vi "Set Output Voltage.vi"(8 "Error In":errorcluster, 9 "Channel":i32, 10 "Voltage":dbl[unit], 11 "BNT_DAQmx-MCSV in":refnum<class "BNT_DAQmx-MCSV.lvclass">) -> (0 "Error Out":errorcluster, 3 "BNT_DAQmx-MCSV out":refnum<class "BNT_DAQmx-MCSV.lvclass">)   [LabVIEW 2016, in "BNT_DAQmx.lvlib" / "BNT_DAQmx-MCSV.lvclass"]
doc: "Write voltage values to DAQmx device and publish.\n\nTimeout is set to constant 1s."
uses:
  BNT_DAQmx-MCSV.lvclass
  BNT_DAQmx-MCSV.lvclass/BNT_DAQmx-MCSV.ctl
  CSPP_Core/Classes/CS++ProcessVariables/PVConnection/PVConnection.lvclass/PVConnection.ctl
  CSPP_Core/Classes/CS++ProcessVariables/ProcessVariable/PV.lvclass/PV.ctl
  <vilib>/DAQmx/write.llb/DAQmx Write (Analog 1D DBL NChan 1Samp).vi
  CSPP_Core/Classes/CS++ProcessVariables/ProcessVariable/Write Data.vi
  CSPP_Core/Classes/CS++ProcessVariables/ProcessVariable/Write Error.vi
  CSPP_Core/Classes/CS++ProcessVariables/ProcessVariable/Write Quality.vi
  CSPP_Core/Classes/CS++ProcessVariables/ProcessVariable/Write status.vi
  CSPP_Core/Classes/CS++ProcessVariables/ProcessVariable/Write Timestamp.vi
  <vilib>/DAQmx/miscellaneous.llb/DAQmx Fill In Error Info.vi
  CSPP_Core/Classes/CS++ProcessVariables/ProcessVariable/PV.lvclass
  CSPP_Core/Classes/CS++ProcessVariables/PVConnection/PVConnection.lvclass
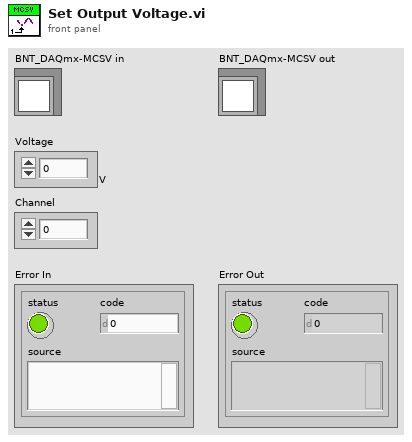
[diagram p1: front panel]
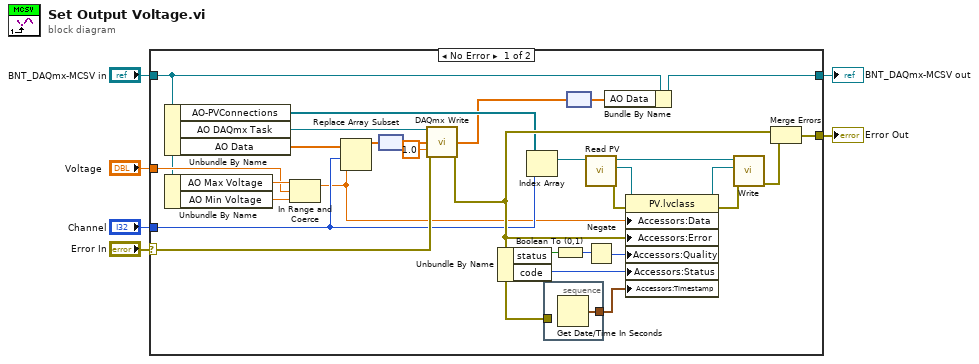
[diagram p0: block diagram]
diagram:
  n1 = case shown="No Error" "Error In" {
    selector: "Error In" -> [w33 w38]
    tunnel: [w25 w38] -> w5
    tunnel: [w17 w37] -> w3
    tunnel: "BNT_DAQmx-MCSV in" -> [w18 w37]
    tunnel: "Voltage" -> [w21 _]
    tunnel: "Channel" -> [w8 _]
    frame No Error {
      n2 = Unbundle By Name(w18) -> ("AO-PVConnections"=w24:refnum<class "PVConnection.lvclass">[], "AO DAQmx Task"=w35:refnum<k21>, "AO Data"=w16:dbl[unit][])
      n3 = Unbundle By Name(w18) -> ("AO Max Voltage"=w23:dbl[unit], "AO Min Voltage"=w22:dbl[unit])
      n4 = In Range and Coerce(upper limit=w23, x=w21, lower limit=w22) -> (coerced(x)=w7:dbl[unit])  [unwired: 1 out]
      n5 = Replace Array Subset(array=w16, new element=w7, index=w8) -> (w15:dbl[unit][])
      n6 = node(w15) -> (w20:dbl[])
      n7 = call-poly <vilib>:"DAQmx Write.vi"("task/channels in"=w35, "data"=w20, "timeout"=1.0, "error in"=w33) -> ("error out"=w26:errorcluster)  [unwired: 9 in, 2 out]
      n8 = Unbundle By Name(w26) -> ("status"=w28:bool, "code"=w31:i32)
      n9 = Index Array(array=w24, index=w8) -> (element=w14:refnum<class "PVConnection.lvclass">)
      n10 = stacked-sequence {
        tunnel: [w36] -> w32
        tunnel: w26 -> [_]
        frame #0 {
          n11 = Get Date/Time In Seconds() -> (seconds since 1Jan1904=w36:timestamp)
        }
      }
      n12 = Boolean To (0,1)(Boolean=w28) -> (0, 1=w29:i16)
      n13 = node(w20) -> (w19:dbl[unit][])
      n14 = call "Read PV.vi"("PVConnection in"=w14) -> ("error out"=w9:errorcluster, "PV"=w10:refnum<class "PV.lvclass">, "PVConnection out"=w11:refnum<class "PVConnection.lvclass">)  [unwired: 8 in]
      n15 = Negate(x=w29) -> (-x=w30:i16)
      n16 = Bundle By Name(cluster=w18, "AO Data"=w19) -> (w17:refnum<class "BNT_DAQmx-MCSV.lvclass">)
      n17 = property class="PV.lvclass"(reference=w10, error in=w9, "Accessors:Data"=w7, "Accessors:Error"=w26, "Accessors:Quality"=w30, "Accessors:Status"=w31, "Accessors:Timestamp"=w32) -> (reference out=w13:refnum<class "PV.lvclass">, error out=w12:errorcluster)
      n18 = call "Write.vi"("error in (no error)"=w12, "PV"=w13, "PVConnection in"=w11) -> ("error out"=w27:errorcluster)  [unwired: 7 in, 1 out]
      n19 = Merge Errors(w26, w27) -> (w25:errorcluster)
    }
    frame Error {
    }
  }
  "Error Out" <- w5
  "BNT_DAQmx-MCSV out" <- w3
